vi "参数设置页.vi"() -> ()   [LabVIEW 2016, in "斯坦道CODcr.lvlib"]
uses:
  <vilib>/Plasmionique/MB Master/MB_Master/MB_Master.lvclass
  <vilib>/ptbypt/NI_PtbyPt.lvlib
panel:
  in  "标样核查自动补测":bool caption="通讯连接"
  in  "跨度核查自动补测":bool caption="通讯连接"
  in  "零点核查自动补测":bool caption="通讯连接"
  in  "标样核查标液偏差":dbl caption="标样核查标液偏差："
  in  "跨度核查标液偏差":dbl caption="跨度核查标液偏差："
  in  "零点核查标液偏差":dbl caption="零点核查标液偏差："
  out "低量程上限":dbl caption="低量程上限："
  in  "简易流程路径":path=path "data/流程.xml"
  out "数据刷新时间":string
  in  "通讯连接":bool
  out "MB table":enum32{"Serial", "TCP"}(tab)
  in  "请选择串口:":refnum<visa-resource-name>
  in  "IP":string="127.0.0.1"
  in  "PORT":string="1001"
  in  "通信方式选择":enum16{"串口", "TCP"}(ring)
  in  "盐度自动补偿：":bool
  out "盐度补偿值":dbl caption="盐度补偿值："
  in  "刷新":bool
  in  "测量模式":T1(ring)
  in  "参数下拉列表":u16(ring)
  in  "量程下拉列表":enum16{"低量程", "高量程"}(ring)
  in  "测试流程路径":path=path "data/流程.xml"
  in  "标样核查量程模式":enum16{"高量程", "低量程", "自动"}(ring) caption="标样核查量程模式："
  in  "加标回收量程模式":enum16{"高量程", "低量程", "自动"}(ring) caption="加标回收量程模式："
  in  "跨度核查量程模式":enum16{"高量程", "低量程", "自动"}(ring) caption="跨度核查量程模式："
  in  "零点核查量程模式":enum16{"高量程", "低量程", "自动"}(ring) caption="零点核查量程模式："
  in  "水样测试量程模式":enum16{"高量程", "低量程", "自动"}(ring) caption="水样测试量程模式："
  out "稀释度":dbl caption="稀释度："
  out "阈值（高->低）":dbl caption="阈值（高->低）："
  out "阈值（低->高）":dbl caption="阈值（低->高）："
  out "量程下限":dbl caption="量程下限："
  out "高量程上限":dbl caption="高量程上限："
  out "检出限":dbl caption="检出限："
  out "曲线截距":dbl caption="曲线截距：" format="%#.6f"
  out "曲线斜率":dbl caption="曲线斜率：" format="%#.6f"
  out "二次多项式系数":dbl caption="二次多项式系数：" format="%#.6f"
  out "消解时长":dbl caption="消解时长："
  out "消解温度":dbl caption="消解温度："
  out "测量精度":u16 caption="测量精度："
  in  "标样核查标液浓度":dbl caption="标样核查标液浓度："
  in  "跨度核查标液浓度":dbl caption="跨度核查标液浓度："
  in  "零点核查标液浓度":dbl caption="零点核查标液浓度："
  in  "跨度值":dbl caption="跨度值："
  # "日质控自动补测设置"
  # "mg/L"
  # "mg/L"
  # "±"
  # "mg/L"
  # "%"
  # "mg/L"
  # "%"
  # "mg/L"
  # "ppt"
  # "mg/L"
  # "mg/L"
  # "mg/L"
  # "mg/L"
  # "mg/L"
  # "min"
  # "℃"
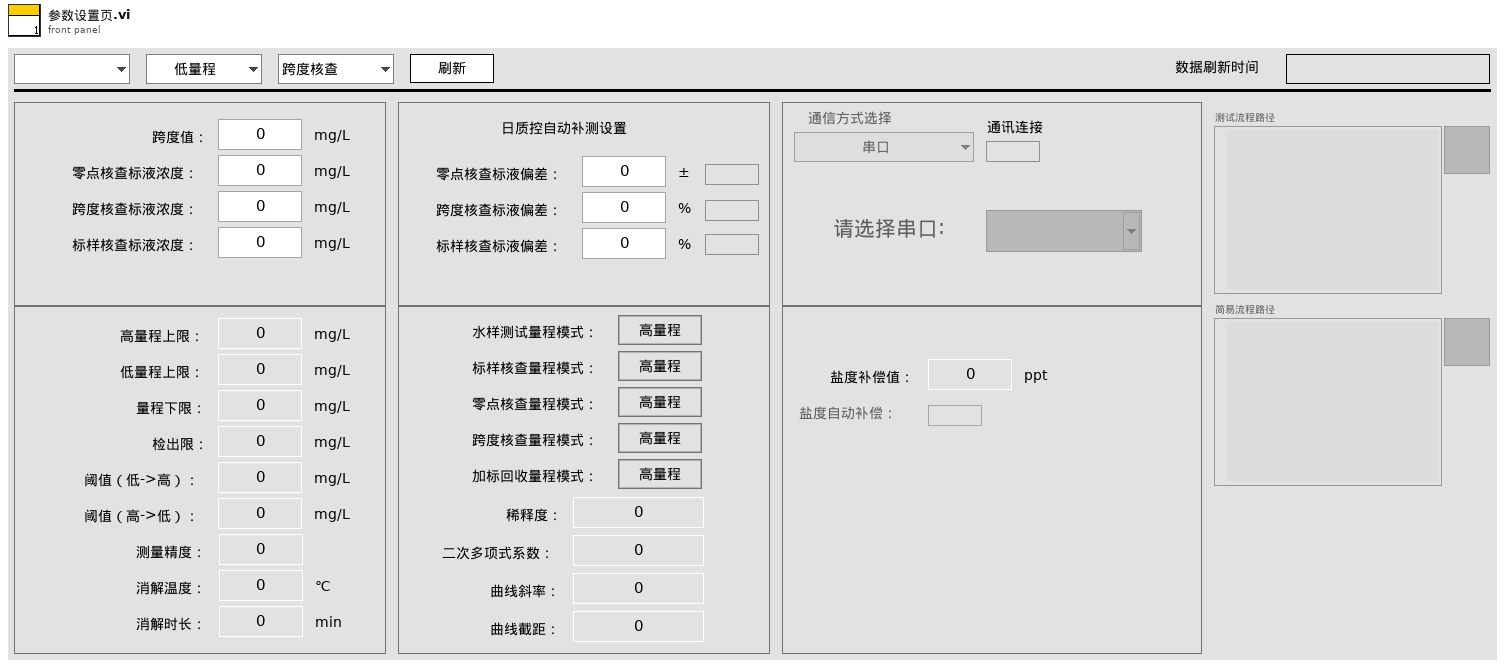
[diagram p1: front panel]
types:
  T1 = enum16{"跨度核查", "水样测量", "零点核查", "标样核查", "加标回收", "快捷测试", "空白校准", "标样校准"}
  T2 = typedef "LVStringsAndValuesArrayTypeDef_U16.ctl" = cluster{"String":string, "Value":u16}[]
  T3 = cluster{"系统时间":timestamp, "工作状态":u16, "测量模式":enum16{"待机", "连续模式", "周期模式", "定点模式", "受控模式", "手动模式"}, "告警代码":u16, "故障代码":u16, "日志代码":u16, "软件版本":u16, "F0":sgl, "F1":sgl, "F2":sgl, "F3":sgl, "T":sgl, "H":sgl, "id":u16, "flowid":u16, "量程":u16, "总磷控温温度1":sgl, "营养盐控温温度2":sgl, "ADC":sgl}
  T4 = enum8{"Enabled", "Disabled", "Disabled and Grayed Out"}
  T5 = cluster{"测量精度":u16, "检出限":dbl, "上限":dbl, "下限":dbl, "阈值（低->高）":dbl, "阈值（高->低）":dbl, "稀释度":dbl}
  T6 = typedef "斯坦道CODcr.lvlib/V3 A版外设参数.ctl" = cluster{"泵类型":u8, "进样速度":u32, "出样速度":u32, "泵阀量":u8, "阀方向":u8, "光谱仪类型":u8, "光谱采样次数":u8, "氙灯次数":u8, "B":u16, "C":u16, "D":u16, "E":u16, "B_COD":u16, "C_COD":u16, "D_COD":u16, "E_COD":u16, "G":u16, "M":u16, "N":u16, "氨氮注射泵控温下限":sgl, "氨氮注射泵控温上限":sgl, "总氮注射泵控温下限":sgl, "总氮注射泵控温上限":sgl, "消解温度下限":sgl, "消解温度上限":sgl, "加热10s限值":sgl, "KP":sgl, "KI":sgl, "KD":sgl, "高温高压阀开阀温度":sgl, "总氮x公式0":u8, "总氮x公式1":sgl, "总氮x公式2":sgl, "总磷浊度稀释系数":sgl, "总磷浊度补偿权重1":sgl, "总磷浊度补偿权重2":sgl, "盐度系数":sgl, "氨氮补偿系数1":sgl, "氨氮补偿系数2":sgl}
  T7 = cluster{"水样测试量程模式":enum16{"高量程", "低量程", "自动"}, "零点核查量程模式":enum16{"高量程", "低量程", "自动"}, "跨度核查量程模式":enum16{"高量程", "低量程", "自动"}, "加标回收量程模式":enum16{"高量程", "低量程", "自动"}, "标样核查量程模式":enum16{"高量程", "低量程", "自动"}}
  T8 = cluster{"总磷跨度值":dbl, "总磷零点标准液浓度":dbl, "总磷跨度标准液浓度":dbl, "总磷标准液标准浓度":dbl, "总氮跨度值":dbl, "总氮零点标准液浓度":dbl, "总氮跨度标准液浓度":dbl, "总氮标准液标准浓度":dbl, "COD跨度值":dbl, "COD零点标准液浓度":dbl, "COD跨度标准液浓度":dbl, "COD标准液标准浓度":dbl, "氨氮跨度值":dbl, "氨氮零点标准液浓度":dbl, "氨氮跨度标准液浓度":dbl, "氨氮标准液标准浓度":dbl, "磷酸盐跨度值":dbl, "磷酸盐零点标准液浓度":dbl, "磷酸盐跨度标准液浓度":dbl, "磷酸盐标准液标准浓度":dbl, "硝氮跨度值":dbl, "硝氮零点标准液浓度":dbl, "硝氮跨度标准液浓度":dbl, "硝氮标准液标准浓度":dbl, "亚硝氮跨度值":dbl, "亚硝氮零点标准液浓度":dbl, "亚硝氮跨度标准液浓度":dbl, "亚硝氮标准液标准浓度":dbl, "硫化物跨度值":dbl, "硫化物零点标准液浓度":dbl, "硫化物跨度标准液浓度":dbl, "硫化物标准液标准浓度":dbl, "硅酸盐跨度值":dbl, "硅酸盐零点标准液浓度":dbl, "硅酸盐跨度标准液浓度":dbl, "硅酸盐标准液标准浓度":dbl, "总磷零点标准液偏差":dbl, "总磷跨度标准液偏差":dbl, "总磷标准液标准偏差":dbl, "总氮零点标准液偏差":dbl, "总氮跨度标准液偏差":dbl, "总氮标准液标准偏差":dbl, "COD零点标准液偏差":dbl, "COD跨度标准液偏差":dbl, "COD标准液标准偏差":dbl, "氨氮零点标准液偏差":dbl, "氨氮跨度标准液偏差":dbl, "氨氮标准液标准偏差":dbl, "磷酸盐零点标准液偏差":dbl, "磷酸盐跨度标准液偏差":dbl, "磷酸盐标准液标准偏差":dbl, "硝氮零点标准液偏差":dbl, "硝氮跨度标准液偏差":dbl, "硝氮标准液标准偏差":dbl, "亚硝氮零点标准液偏差":dbl, "亚硝氮跨度标准液偏差":dbl, "亚硝氮标准液标准偏差":dbl, "硫化物零点标准液偏差":dbl, "硫化物跨度标准液偏差":dbl, "硫化物标准液标准偏差":dbl, "硅酸盐零点标准液偏差":dbl, "硅酸盐跨度标准液偏差":dbl, "硅酸盐标准液标准偏差":dbl, "氟化物跨度值":dbl, "氟化物零点标准液浓度":dbl, "氟化物跨度标准液浓度":dbl, "氟化物标准液标准浓度":dbl, "氟化物零点标准液偏差":dbl, "氟化物跨度标准液偏差":dbl, "氟化物标准液标准偏差":dbl}
  T9 = cluster{"总磷":dbl, "总氮":dbl, "氨氮":dbl, "磷酸盐":dbl, "硝氮":dbl, "亚硝氮":dbl, "硅酸盐":dbl, "硫化物":dbl, "COD":dbl, "氟化物":dbl}
  T10 = cluster{"水样测试量程模式":u16, "零点核查量程模式":u16, "跨度核查量程模式":u16, "加标回收量程模式":u16, "标样核查量程模式":u16}
  T11 = cluster{"水样测试量程模式":enum16{"H", "L", "AUTO"}, "空白核查量程模式":enum16{"H", "L", "AUTO"}, "跨度核查量程模式":enum16{"H", "L", "AUTO"}, "加标回收量程模式":enum16{"H", "L", "AUTO"}, "标样核查量程模式":enum16{"H", "L", "AUTO"}}
  T12 = cluster{"水样测试量程模式":u16, "空白核查量程模式":u16, "跨度核查量程模式":u16, "加标回收量程模式":u16, "标样核查量程模式":u16}
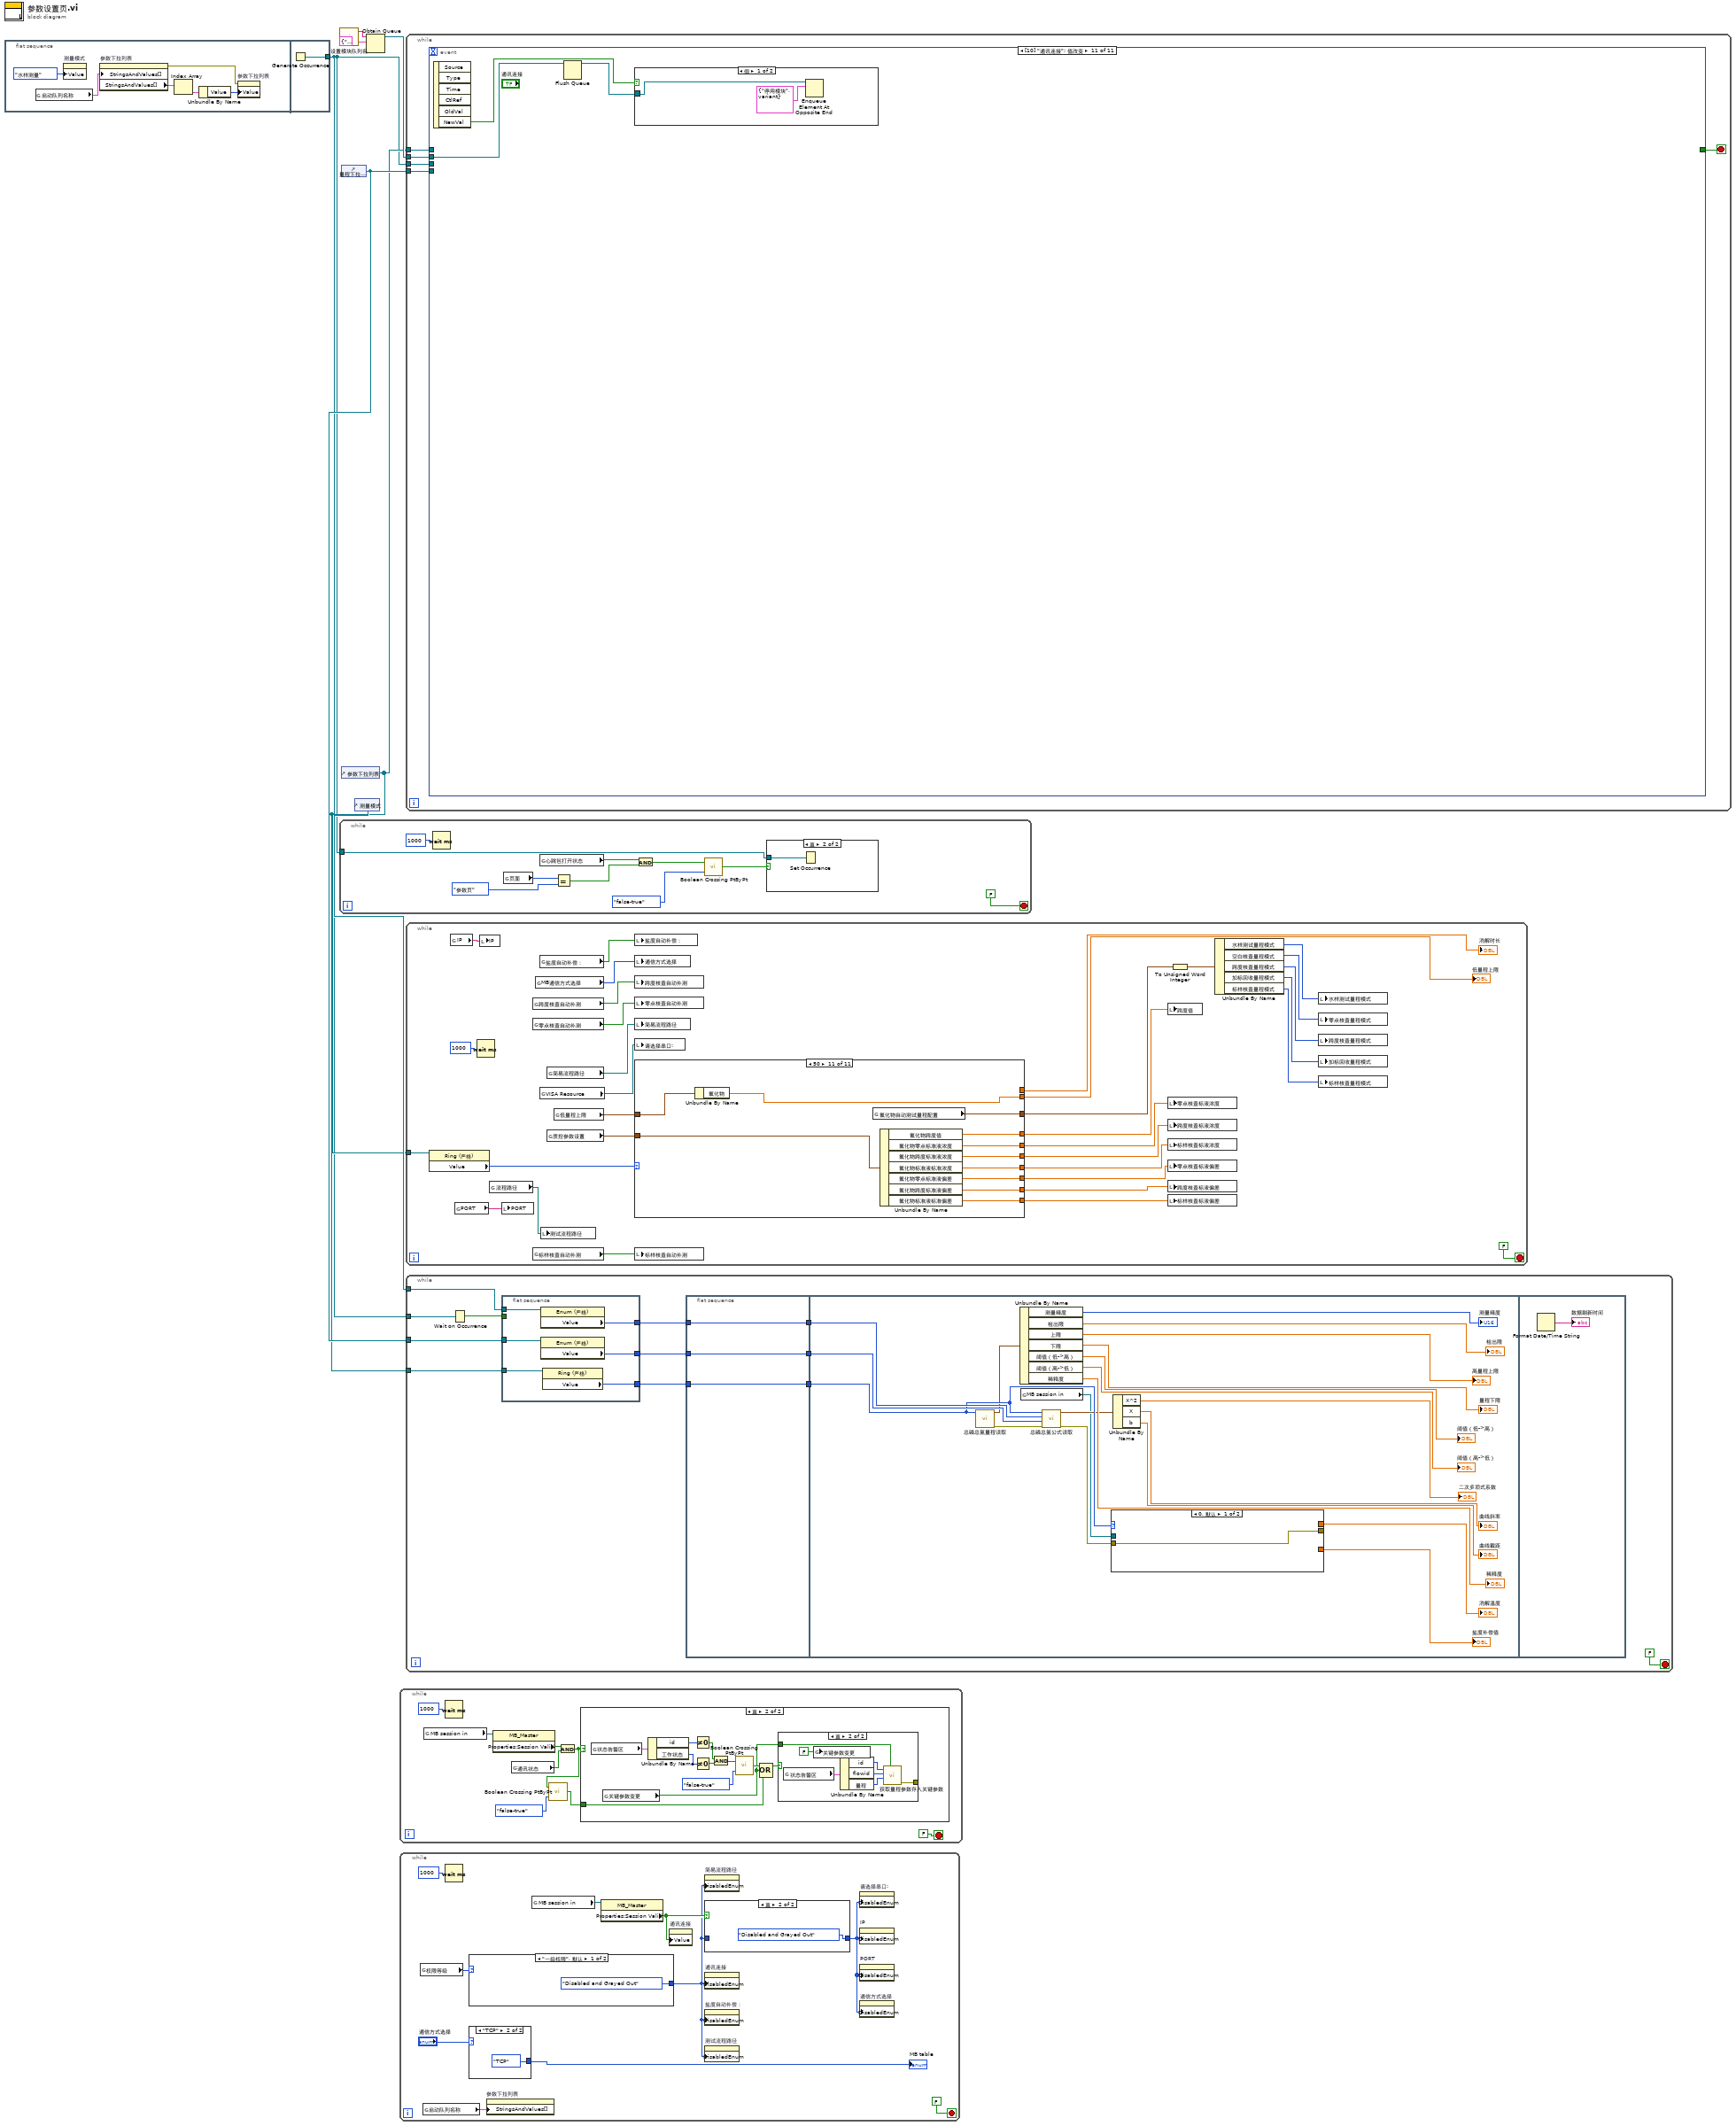
[diagram p0: block diagram]
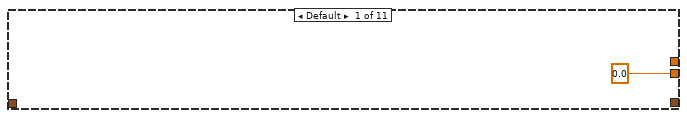
[diagram p5: hidden frame]
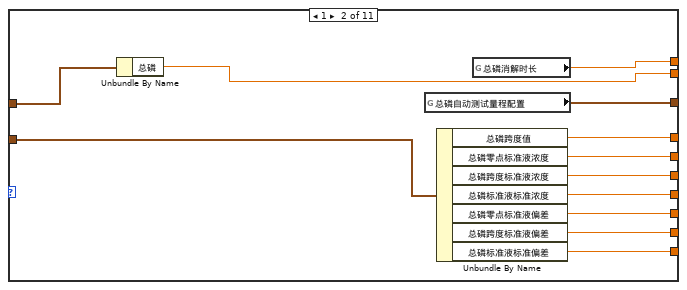
[diagram p6: hidden frame]
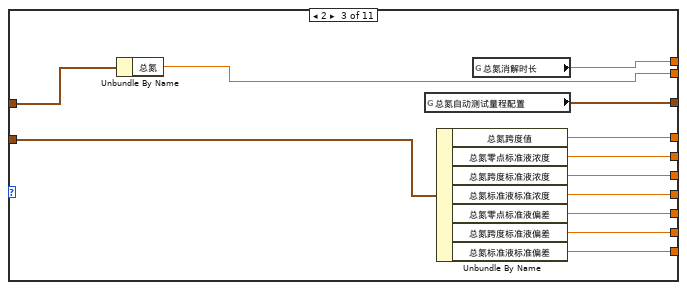
[diagram p7: hidden frame]
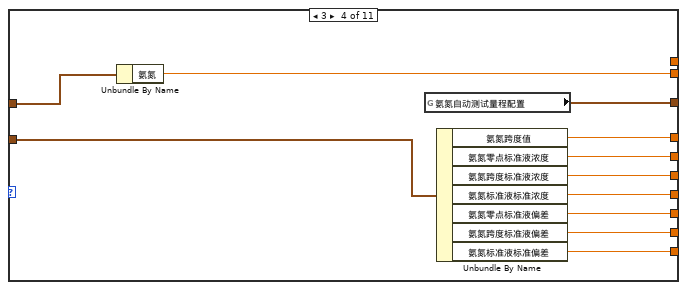
[diagram p8: hidden frame]
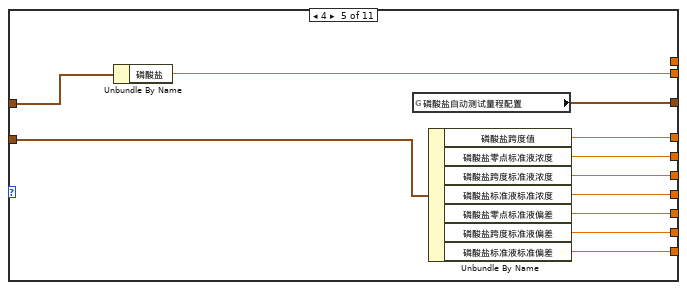
[diagram p9: hidden frame]
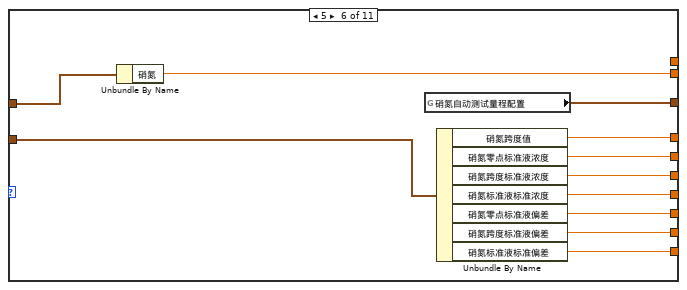
[diagram p10: hidden frame]
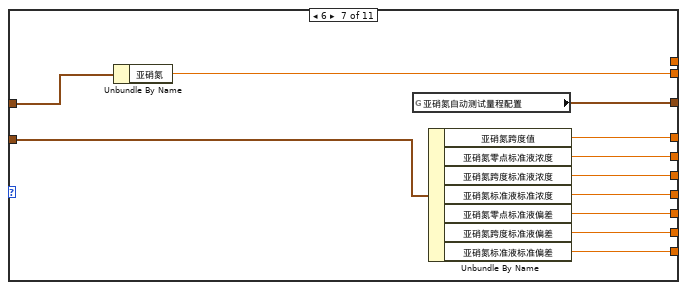
[diagram p11: hidden frame]
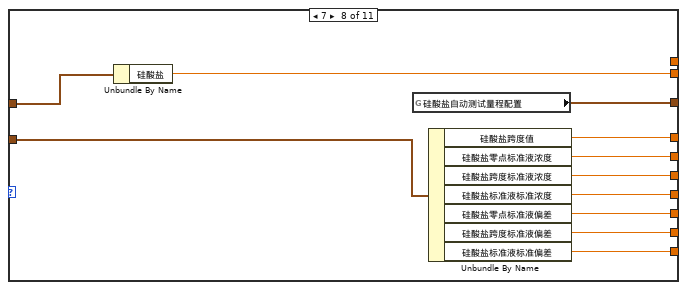
[diagram p12: hidden frame]
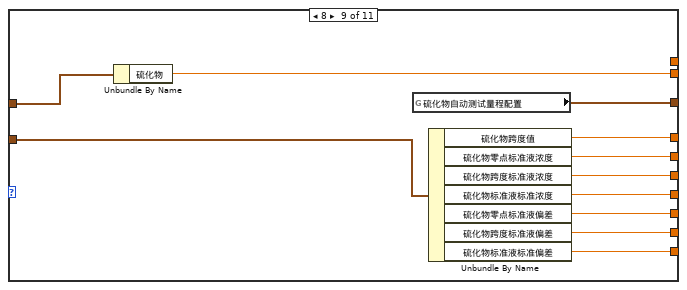
[diagram p13: hidden frame]
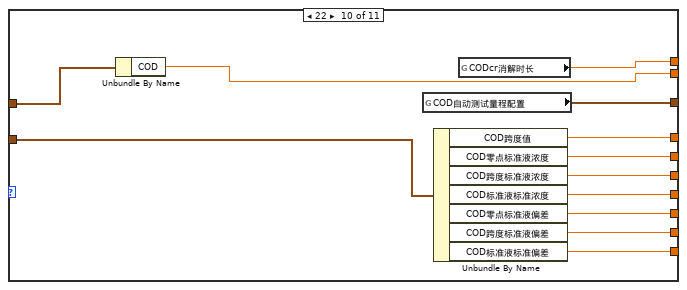
[diagram p14: hidden frame]
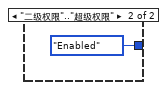
[diagram p15: hidden frame]
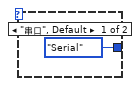
[diagram p16: hidden frame]
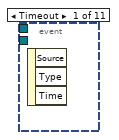
[diagram p18: hidden frame]
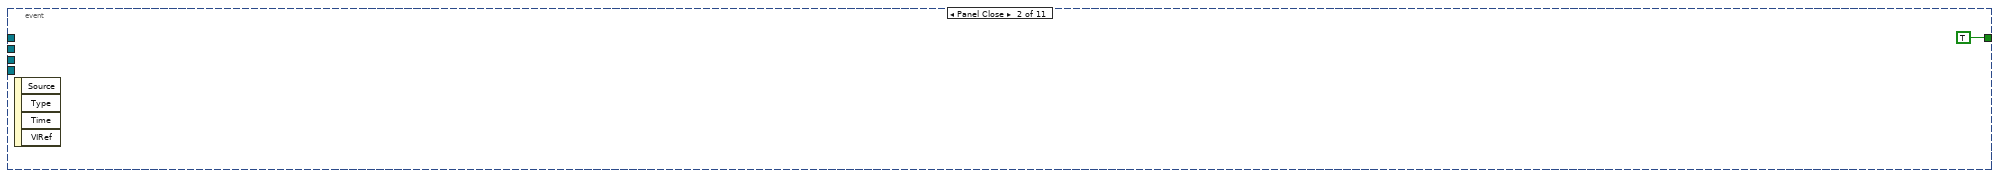
[diagram p19: hidden frame]
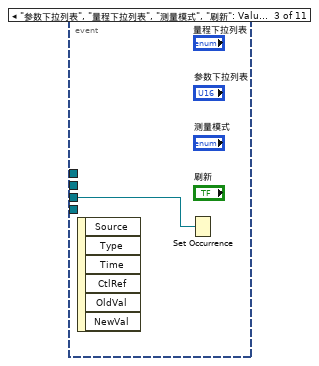
[diagram p20: hidden frame]
diagram:
  n1 = flat-sequence {
    tunnel: [w14] -> w1
    frame #0 {
      n2 = global read "model config var.vi" "启动队列名称"() -> (w9:cluster{"String":string, "Value":u16}[])
      n3 = property on="测量模式" class="Enum (严格)"("Value"=T1."水样测量" ("测量模式")) -> ()  [unwired: 2 in, 2 out]
      n4 = property on="参数下拉列表" class="Ring (严格)"("StringsAndValues[]"=w9) -> (error out=w12:errorcluster, "StringsAndValues[]"=w10:T2)  [unwired: 2 in, 1 out]
      n5 = Index Array(array=w10) -> (element=w11:cluster{"String":string, "Value":u16})  [unwired: 1 in]
      n6 = Unbundle By Name(w11) -> ("Value"=w13:u16)
      n7 = property on="参数下拉列表" class="Ring (严格)"(error in=w12, "Value"=w13) -> ()  [unwired: 1 in, 2 out]
    }
    frame #1 {
      n8 = Generate Occurrence() -> (w14:refnum<k4>)
    }
  }
  n9 = call "设置模块队列名.vi"() -> ("Msg"=w6:string)  [unwired: 5 in]
  n10 = while {
    tunnel: w1 -> [w21]
    stop <- FALSE stop-if-true
    n11 = Wait (ms)(milliseconds to wait=u32 1000 ("等待时间（毫秒）")) -> ()  [unwired: 1 out]
    n12 = global read "VAR总磷总氮全局变量.vi" "页面"() -> (w23:enum16{"主页", "参数页", "校准页"})
    n13 = global read "VAR总磷总氮全局变量.vi" "心跳包打开状态"() -> (w17:bool)
    n14 = Equal?(x=w23, y=enum16{"主页", "参数页", "校准页"}."参数页" ("页面")) -> (x = y?=w22:bool)
    n15 = And(x=w17, y=w22) -> (x .and. y?=w18:bool)
    n16 = call <vilib>:"Boolean Crossing PtByPt.vi"("direction"=enum16{"either", "false-true", "true-false"}."false-true", "input"=w18) -> ("crossing"=w16:bool)  [unwired: 1 in]
    n17 = case shown="真" w16 {
      tunnel: w21 -> [_ w25]
      frame False {
      }
      frame True {
        n18 = Set Occurrence(w25) -> ()
      }
    }
  }
  n19 = control-ref of="量程下拉列表"() -> (w3:refnum<vi>)
  n20 = control-ref of="参数下拉列表"() -> (w2:refnum<vi>)
  n21 = control-ref of="测量模式"() -> (w4:refnum<vi>)
  n22 = Obtain Queue(name (unnamed)=w6, element data type=cluster{"命令":string, "data":variant} {"命令"="", "data"=variant}) -> (queue out=w5:refnum<queue>)  [unwired: 3 in, 2 out]
  n23 = while {
    stop <- FALSE stop-if-true
    n24 = global read "VAR总磷总氮全局变量.vi" "MB session in"() -> (w30:refnum<class "MB_Master.lvclass">)
    n25 = Wait (ms)(milliseconds to wait=u32 1000 ("等待时间（毫秒）")) -> ()  [unwired: 1 out]
    n26 = property class="MB_Master"(reference=w30) -> ("Properties:Session Valid"=w29:bool)  [unwired: 1 in, 2 out]
    n27 = global read "VAR总磷总氮全局变量.vi" "通讯状态"() -> (w32:bool)
    n28 = And(x=w29, y=w32) -> (x .and. y?=w27:bool)
    n29 = call <vilib>:"Boolean Crossing PtByPt.vi"("direction"=enum16{"either", "false-true", "true-false"}."false-true", "input"=w27) -> ("crossing"=w26:bool)  [unwired: 1 in]
    n30 = case shown="真" w27 {
      tunnel: w26 -> [_ w34]
      frame False {
      }
      frame True {
        n31 = global read "VAR总磷总氮全局变量.vi" "状态告警区"() -> (w44:T3)
        n32 = global read "VAR总磷总氮全局变量.vi" "关键参数变更"() -> (w35:bool)
        n33 = Unbundle By Name(w44) -> ("id"=w38:u16, "工作状态"=w43:u16)
        n34 = Not Equal To 0?(x=w38) -> (x != 0?=w39:bool)
        n35 = Not Equal To 0?(x=w43) -> (x != 0?=w40:bool)
        n36 = And(x=w39, y=w40) -> (x .and. y?=w41:bool)
        n37 = call <vilib>:"Boolean Crossing PtByPt.vi"("direction"=enum16{"either", "false-true", "true-false"}."false-true", "input"=w41) -> ("crossing"=w37:bool)  [unwired: 1 in]
        n38 = Compound Arithmetic op=OR ("复合运算")(w37, w35, w34) -> (w36:bool)
        n39 = case shown="真" w36 {
          tunnel: [_ w51] -> _
          tunnel: w35 -> [_ w46]
          frame False {
          }
          frame True {
            n40 = global read "VAR总磷总氮全局变量.vi" "状态告警区"() -> (w50:T3)
            n41 = global write "VAR总磷总氮全局变量.vi" "关键参数变更"(FALSE ("关键参数变更")) -> ()
            n42 = Unbundle By Name(w50) -> ("id"=w49:u16, "flowid"=w48:u16, "量程"=w47:u16)
            n43 = call "获取量程参数存入关键参数.vi"("关键参数变更"=w46, "量程"=w47, "flowid"=w48, "id"=w49) -> ("error out"=w51:errorcluster)  [unwired: 7 in]
          }
        }
      }
    }
  }
  n44 = while {
    stop <- FALSE stop-if-true
    n45 = global read "VAR总磷总氮全局变量.vi" "权限等级"() -> (w54:enum16{"一级权限", "二级权限", "三级权限", "超级权限"})
    n46 = global read "model config var.vi" "启动队列名称"() -> (w52:cluster{"String":string, "Value":u16}[])
    n47 = Wait (ms)(milliseconds to wait=u32 1000 ("等待时间（毫秒）")) -> ()  [unwired: 1 out]
    n48 = case shown="\"一级权限\", 默认" w54 {
      tunnel: [T4."Disabled and Grayed Out" ("禁用") T4."Enabled" ("禁用")] -> w53
      frame "一级权限", Default {
      }
      frame "二级权限".."超级权限" {
      }
    }
    n49 = case shown="\"TCP\"" "通信方式选择" {
      tunnel: [enum32{"Serial", "TCP"}."Serial" ("MB table") enum32{"Serial", "TCP"}."TCP" ("MB table")] -> w56
      frame "串口", Default {
      }
      frame "TCP" {
      }
    }
    "MB table" <- w56
    n50 = property on="参数下拉列表" class="Ring (严格)"("StringsAndValues[]"=w52) -> ()  [unwired: 2 in, 2 out]
    n51 = global read "VAR总磷总氮全局变量.vi" "MB session in"() -> (w60:refnum<class "MB_Master.lvclass">)
    n52 = property class="MB_Master"(reference=w60) -> ("Properties:Session Valid"=w58:bool)  [unwired: 1 in, 2 out]
    n53 = property on="通讯连接" class="Bool (严格)"("Value"=w58) -> ()  [unwired: 2 in, 2 out]
    n54 = property on="简易流程路径" class="Path"("DisabledEnum"=w53) -> ()  [unwired: 2 in, 2 out]
    n55 = case shown="真" w58 {
      tunnel: [w66 T4."Disabled and Grayed Out" ("禁用")] -> w57
      tunnel: w53 -> [w66 _]
      frame False {
      }
      frame True {
      }
    }
    n56 = property on="通讯连接" class="Bool (严格)"("DisabledEnum"=w53) -> ()  [unwired: 2 in, 2 out]
    n57 = property on="盐度自动补偿：" class="Bool (严格)"("DisabledEnum"=w53) -> ()  [unwired: 2 in, 2 out]
    n58 = property on="测试流程路径" class="Path"("DisabledEnum"=w53) -> ()  [unwired: 2 in, 2 out]
    n59 = property on="请选择串口:" class="VISAName"("DisabledEnum"=w57) -> ()  [unwired: 2 in, 2 out]
    n60 = property on="IP" class="Str"("DisabledEnum"=w57) -> ()  [unwired: 2 in, 2 out]
    n61 = property on="PORT" class="Str"("DisabledEnum"=w57) -> ()  [unwired: 2 in, 2 out]
    n62 = property on="通信方式选择" class="Enum (严格)"("DisabledEnum"=w57) -> ()  [unwired: 2 in, 2 out]
  }
  n63 = while {
    tunnel: w1 -> [w71]
    tunnel: w2 -> [w70]
    tunnel: w5 -> [w69]
    tunnel: w3 -> [w68]
    stop <- w72 stop-if-true
    n64 = event shown="[10] \"通讯连接\": 值改变" {
      selector: _ -> [_ _ _ _ _ _ _ _ _ _ _]
      dyn-events: _ -> [_ _ _ _ _ _ _ _ _ _ _]
      timeout: _ -> [_ _ _ _ _ _ _ _ _ _ _]
      tunnel: [_ TRUE _ _ _ _ _ _ _ _ _] -> w72
      tunnel: w71 -> [_ _ w74 _ _ _ _ _ _ w122 _]
      tunnel: w70 -> [_ _ _ _ w93 _ _ _ _ w124 _]
      tunnel: w69 -> [_ _ _ _ _ _ _ _ _ _ w293]
      tunnel: w68 -> [_ _ _ _ _ _ _ _ _ _ _]
      event Timeout {
        n65 = event-data() -> ()  [unwired: 1 in, 3 out]
      }
      event Panel Close {
        n66 = event-data() -> ()  [unwired: 1 in, 4 out]
      }
      event "参数下拉列表", "量程下拉列表", "测量模式", "刷新": Value Change {
        n67 = event-data() -> ()  [unwired: 1 in, 6 out]
        n68 = Set Occurrence(w74) -> ()
      }
      event "跨度值", "零点核查标液浓度", "跨度核查标液浓度", "标样核查标液浓度", "消解温度", "消解时长", "检出限", "高量程上限", "量程下限", "阈值（低->高）", "阈值（高->低）", "稀释度", "低量程上限", "零点核查标液偏差", "跨度核查标液偏差", "标样核查标液偏差": Mouse Down {
        n69 = event-data() -> ("CtlRef"=w76:refnum<vi>)  [unwired: 1 in, 5 out]
        n70 = global read "VAR总磷总氮全局变量.vi" "权限等级"() -> (w75:enum16{"一级权限", "二级权限", "三级权限", "超级权限"})
        n71 = case shown="\"二级权限\"..\"超级权限\"" w75 {
          tunnel: w76 -> [_ w80]
          frame "一级权限", Default {
          }
          frame "二级权限".."超级权限" {
            n72 = property class="DigNum (严格)"(reference=w80) -> (reference out=w78:refnum<vi>, "Value"=w79:dbl)  [unwired: 1 in, 1 out]
            n73 = call "数字键盘.vi"("OldNumber"=w79) -> ("NewNumber"=w77:dbl)
            n74 = property class="DigNum (严格)"(reference=w78, "Val(Sgnl)"=w77) -> ()  [unwired: 1 in, 2 out]
          }
        }
      }
      event "测量精度", "检出限", "高量程上限", "量程下限", "阈值（低->高）", "阈值（高->低）", "稀释度": Value Change {
        n75 = event-data() -> ()  [unwired: 1 in, 6 out]
        n76 = property class="Ring (严格)"(reference=w93) -> ("Value"=w92:u16)  [unwired: 1 in, 2 out]
        n77 = local read "阈值（低->高）"() -> (w86:dbl)
        n78 = local read "阈值（高->低）"() -> (w85:dbl)
        n79 = local read "高量程上限"() -> (w89:dbl)
        n80 = local read "测量精度"() -> (w83:u16)
        n81 = local read "量程下限"() -> (w88:dbl)
        n82 = local read "检出限"() -> (w87:dbl)
        n83 = local read "稀释度"() -> (w84:dbl)
        n84 = Bundle By Name(cluster=T5 {"测量精度"=0, "检出限"=0.0, "上限"=0.0, "下限"=0.0, "阈值（低->高）"=0.0, "阈值（高->低）"=0.0, "稀释度"=0.0} ("量程参数写入"), "测量精度"=w83, "检出限"=w87, "上限"=w89, "下限"=w88, "阈值（低->高）"=w86, "阈值（高->低）"=w85, "稀释度"=w84) -> (w90:T5)
        n85 = call "总磷总氮量程写入.vi"("量程参数写入"=w90, "测量参数"=w92) -> ("error out"=w81:errorcluster)  [unwired: 8 in]
        n86 = case shown="无错误" w81 {
          tunnel: ["写入成功" "写入失败"] -> w82
          frame No Error {
            n87 = global write "VAR总磷总氮全局变量.vi" "关键参数变更"(TRUE ("关键参数变更")) -> ()
          }
          frame Error {
          }
        }
        n88 = One Button Dialog(message=w82) -> ()  [unwired: 1 in, 1 out]
      }
      event "消解温度": Value Change {
        n89 = event-data() -> ("NewVal"=w99:dbl)  [unwired: 1 in, 5 out]
        n90 = global read "VAR总磷总氮全局变量.vi" "MB session in"() -> (w100:refnum<class "MB_Master.lvclass">)
        n91 = call "读取外设配置.vi"("MB session in"=w100) -> ("error out"=w103:errorcluster, "外设配置"=w102:T6)  [unwired: 8 in, 1 out]
        n92 = Bundle By Name(cluster=w102, "消解温度下限"=w99) -> (w101:T6)
        n93 = call "写入外设配置.vi"("error in (no error)"=w103, "外设配置"=w101, "MB session in"=w100) -> ("error out"=w98:errorcluster)  [unwired: 7 in, 1 out]
        n94 = case shown="错误" w98 {
          tunnel: ["写入成功" "写入失败"] -> w97
          frame No Error {
          }
          frame Error {
          }
        }
        n95 = One Button Dialog(message=w97) -> ()  [unwired: 1 in, 1 out]
      }
      event "测量精度": Mouse Down {
        n96 = event-data() -> ("CtlRef"=w107:refnum<vi>)  [unwired: 1 in, 7 out]
        n97 = global read "VAR总磷总氮全局变量.vi" "权限等级"() -> (w106:enum16{"一级权限", "二级权限", "三级权限", "超级权限"})
        n98 = case shown="\"二级权限\"..\"超级权限\"" w106 {
          tunnel: w107 -> [_ w111]
          frame "一级权限", Default {
          }
          frame "二级权限".."超级权限" {
            n99 = property class="DigNum (严格)"(reference=w111) -> (reference out=w109:refnum<vi>, "Value"=w110:u16)  [unwired: 1 in, 1 out]
            n100 = call "数字键盘.vi"("OldNumber"=w110) -> ("NewNumber"=w108:dbl)
            n101 = property class="DigNum (严格)"(reference=w109, "Val(Sgnl)"=w108) -> ()  [unwired: 1 in, 2 out]
          }
        }
      }
      event "盐度补偿值": Mouse Down {
        n102 = event-data() -> ("CtlRef"=w113:refnum<vi>)  [unwired: 1 in, 3 out]
        n103 = global read "VAR总磷总氮全局变量.vi" "权限等级"() -> (w112:enum16{"一级权限", "二级权限", "三级权限", "超级权限"})
        n104 = case shown="\"二级权限\"..\"超级权限\"" w112 {
          tunnel: w113 -> [_ w115]
          frame "一级权限", Default {
          }
          frame "二级权限".."超级权限" {
            n105 = case shown="假" "盐度自动补偿：" {
              tunnel: w115 -> [w119 _]
              frame False {
                n106 = property class="DigNum (严格)"(reference=w119) -> (reference out=w117:refnum<vi>, "Value"=w118:dbl)  [unwired: 1 in, 1 out]
                n107 = call "数字键盘.vi"("OldNumber"=w118) -> ("NewNumber"=w116:dbl)
                n108 = property class="DigNum (严格)"(reference=w117, "Val(Sgnl)"=w116) -> ()  [unwired: 1 in, 2 out]
              }
              frame True {
              }
            }
          }
        }
      }
      event "盐度补偿值": Value Change {
        n109 = event-data() -> ("NewVal"=w120:dbl)  [unwired: 1 in, 5 out]
        n110 = global read "VAR总磷总氮全局变量.vi" "MB session in"() -> (w121:refnum<class "MB_Master.lvclass">)
        n111 = call "盐度补偿值写入.vi"("盐度补偿值"=w120, "MB session in"=w121) -> ()  [unwired: 8 in, 2 out]
      }
      event "跨度值", "零点核查标液浓度", "跨度核查标液浓度", "标样核查标液浓度", "消解时长", "水样测试量程模式", "零点核查量程模式", "跨度核查量程模式", "加标回收量程模式", "标样核查量程模式", "测试流程路径", "盐度自动补偿：", "IP", "PORT", "请选择串口:", "通信方式选择", "简易流程路径", "低量程上限", "零点核查标液偏差", "跨度核查标液偏差", "标样核查标液偏差", "零点核查自动补测", "跨度核查自动补测", "标样核查自动补测": Value Change {
        n112 = event-data() -> ()  [unwired: 1 in, 6 out]
        n113 = global read "VAR总磷总氮全局变量.vi" "权限等级"() -> (w123:enum16{"一级权限", "二级权限", "三级权限", "超级权限"})
        n114 = case shown="\"二级权限\"..\"超级权限\"" w123 {
          tunnel: w124 -> [_ w126]
          tunnel: w122 -> [w125 _]
          frame "一级权限", Default {
            n115 = Set Occurrence(w125) -> ()
          }
          frame "二级权限".."超级权限" {
            n116 = flat-sequence {
              tunnel: w126 -> [w156]
              frame #0 {
                n117 = property class="Ring (严格)"(reference=w156) -> ("Value"=w155:u16)  [unwired: 1 in, 2 out]
                n118 = global write "总磷总氮断电保存全局变量.vi" "IP"("IP") -> ()
                n119 = global write "总磷总氮断电保存全局变量.vi" "PORT"("PORT") -> ()
                n120 = local read "盐度自动补偿："() -> (w142:bool)
                n121 = local read "通信方式选择"() -> (w138:enum16{"串口", "TCP"})
                n122 = global write "总磷总氮断电保存全局变量.vi" "流程路径"("测试流程路径") -> ()
                n123 = global write "总磷总氮断电保存全局变量.vi" "简易流程路径"("简易流程路径") -> ()
                n124 = global write "总磷总氮断电保存全局变量.vi" "VISA Resource"("请选择串口:") -> ()
                n125 = global write "总磷总氮断电保存全局变量.vi" "MB通信方式选择"(w138) -> ()
                n126 = global write "总磷总氮断电保存全局变量.vi" "盐度自动补偿："(w142) -> ()
                n127 = global write "总磷总氮断电保存全局变量.vi" "标样核查自动补测"("标样核查自动补测") -> ()
                n128 = global write "总磷总氮断电保存全局变量.vi" "跨度核查自动补测"("跨度核查自动补测") -> ()
                n129 = global write "总磷总氮断电保存全局变量.vi" "零点核查自动补测"("零点核查自动补测") -> ()
                n130 = Bundle("水样测试量程模式"="水样测试量程模式", "零点核查量程模式"="零点核查量程模式", "跨度核查量程模式"="跨度核查量程模式", "加标回收量程模式"="加标回收量程模式", "标样核查量程模式"="标样核查量程模式") -> (w144:T7)  [unwired: 1 in]
                n131 = global read "总磷总氮断电保存全局变量.vi" "质控参数设置"() -> (w150:T8)
                n132 = global read "总磷总氮断电保存全局变量.vi" "低量程上限"() -> (w135:T9)
                n133 = local read "消解时长"() -> (w137:dbl)
                n134 = property on="低量程上限" class="DigNum (严格)"() -> ("Value"=w133:dbl)  [unwired: 2 in, 2 out]
                n135 = To Unsigned Word Integer(number=w144) -> (unsigned 16bit integer=w143:T10)
                n136 = case shown="50" w155 {
                  tunnel: "跨度值" -> [_ w170 w184 w197 w210 w223 w236 w249 w262 w276 w289]
                  tunnel: "标样核查标液浓度" -> [_ w167 w181 w194 w207 w220 w233 w246 w259 w273 w286]
                  tunnel: "跨度核查标液浓度" -> [_ w168 w182 w195 w208 w221 w234 w247 w260 w274 w287]
                  tunnel: "零点核查标液浓度" -> [_ w169 w183 w196 w209 w222 w235 w248 w261 w275 w288]
                  tunnel: w150 -> [_ w172 w186 w199 w212 w225 w238 w251 w264 w278 w291]
                  tunnel: w143 -> [_ w166 w180 w193 w206 w219 w232 w245 w258 w271 w285]
                  tunnel: w137 -> [_ w165 w179 _ _ _ _ _ _ w272 _]
                  tunnel: w135 -> [w158 w163 w178 w192 w205 w218 w231 w244 w257 w270 w284]
                  tunnel: [w158 w162 w176 w191 w204 w217 w230 w243 w256 w269 w283] -> w134
                  tunnel: w133 -> [_ w164 w177 w190 w203 w216 w229 w242 w255 w268 w282]
                  tunnel: "标样核查标液偏差" -> [_ w161 w173 w187 w200 w215 w226 w239 w252 w265 w279]
                  tunnel: "跨度核查标液偏差" -> [_ w160 w174 w188 w201 w214 w227 w240 w253 w266 w280]
                  tunnel: "零点核查标液偏差" -> [_ w159 w175 w189 w202 w213 w228 w241 w254 w267 w281]
                  frame 0, Default {
                  }
                  frame 1 {
                    n137 = global write "总磷总氮断电保存全局变量.vi" "总磷消解时长"(w165) -> ()
                    n138 = global write "总磷总氮断电保存全局变量.vi" "总磷自动测试量程配置"(w166) -> ()
                    n139 = Bundle By Name(cluster=w172, "总磷跨度值"=w170, "总磷零点标准液浓度"=w169, "总磷跨度标准液浓度"=w168, "总磷标准液标准浓度"=w167, "总磷零点标准液偏差"=w159, "总磷跨度标准液偏差"=w160, "总磷标准液标准偏差"=w161) -> (w171:T8)
                    n140 = Bundle By Name(cluster=w163, "总磷"=w164) -> (w162:T9)
                    n141 = global write "总磷总氮断电保存全局变量.vi" "质控参数设置"(w171) -> ()
                  }
                  frame 2 {
                    n142 = global write "总磷总氮断电保存全局变量.vi" "总氮消解时长"(w179) -> ()
                    n143 = global write "总磷总氮断电保存全局变量.vi" "总氮自动测试量程配置"(w180) -> ()
                    n144 = Bundle By Name(cluster=w186, "总氮跨度值"=w184, "总氮零点标准液浓度"=w183, "总氮跨度标准液浓度"=w182, "总氮标准液标准浓度"=w181, "总氮零点标准液偏差"=w175, "总氮跨度标准液偏差"=w174, "总氮标准液标准偏差"=w173) -> (w185:T8)
                    n145 = Bundle By Name(cluster=w178, "总氮"=w177) -> (w176:T9)
                    n146 = global write "总磷总氮断电保存全局变量.vi" "质控参数设置"(w185) -> ()
                  }
                  frame 3 {
                    n147 = global write "总磷总氮断电保存全局变量.vi" "氨氮自动测试量程配置"(w193) -> ()
                    n148 = Bundle By Name(cluster=w199, "氨氮跨度值"=w197, "氨氮零点标准液浓度"=w196, "氨氮跨度标准液浓度"=w195, "氨氮标准液标准浓度"=w194, "氨氮零点标准液偏差"=w189, "氨氮跨度标准液偏差"=w188, "氨氮标准液标准偏差"=w187) -> (w198:T8)
                    n149 = Bundle By Name(cluster=w192, "氨氮"=w190) -> (w191:T9)
                    n150 = global write "总磷总氮断电保存全局变量.vi" "质控参数设置"(w198) -> ()
                  }
                  frame 4 {
                    n151 = Bundle By Name(cluster=w212, "磷酸盐跨度值"=w210, "磷酸盐零点标准液浓度"=w209, "磷酸盐跨度标准液浓度"=w208, "磷酸盐标准液标准浓度"=w207, "磷酸盐零点标准液偏差"=w202, "磷酸盐跨度标准液偏差"=w201, "磷酸盐标准液标准偏差"=w200) -> (w211:T8)
                    n152 = global write "总磷总氮断电保存全局变量.vi" "磷酸盐自动测试量程配置"(w206) -> ()
                    n153 = Bundle By Name(cluster=w205, "磷酸盐"=w203) -> (w204:T9)
                    n154 = global write "总磷总氮断电保存全局变量.vi" "质控参数设置"(w211) -> ()
                  }
                  frame 5 {
                    n155 = global write "总磷总氮断电保存全局变量.vi" "硝氮自动测试量程配置"(w219) -> ()
                    n156 = Bundle By Name(cluster=w225, "硝氮跨度值"=w223, "硝氮零点标准液浓度"=w222, "硝氮跨度标准液浓度"=w221, "硝氮标准液标准浓度"=w220, "硝氮零点标准液偏差"=w213, "硝氮跨度标准液偏差"=w214, "硝氮标准液标准偏差"=w215) -> (w224:T8)
                    n157 = Bundle By Name(cluster=w218, "硝氮"=w216) -> (w217:T9)
                    n158 = global write "总磷总氮断电保存全局变量.vi" "质控参数设置"(w224) -> ()
                  }
                  frame 6 {
                    n159 = Bundle By Name(cluster=w238, "亚硝氮跨度值"=w236, "亚硝氮零点标准液浓度"=w235, "亚硝氮跨度标准液浓度"=w234, "亚硝氮标准液标准浓度"=w233, "亚硝氮零点标准液偏差"=w228, "亚硝氮跨度标准液偏差"=w227, "亚硝氮标准液标准偏差"=w226) -> (w237:T8)
                    n160 = global write "总磷总氮断电保存全局变量.vi" "亚硝氮自动测试量程配置"(w232) -> ()
                    n161 = Bundle By Name(cluster=w231, "亚硝氮"=w229) -> (w230:T9)
                    n162 = global write "总磷总氮断电保存全局变量.vi" "质控参数设置"(w237) -> ()
                  }
                  frame 7 {
                    n163 = Bundle By Name(cluster=w251, "硅酸盐跨度值"=w249, "硅酸盐零点标准液浓度"=w248, "硅酸盐跨度标准液浓度"=w247, "硅酸盐标准液标准浓度"=w246, "硅酸盐零点标准液偏差"=w241, "硅酸盐跨度标准液偏差"=w240, "硅酸盐标准液标准偏差"=w239) -> (w250:T8)
                    n164 = global write "总磷总氮断电保存全局变量.vi" "硅酸盐自动测试量程配置"(w245) -> ()
                    n165 = Bundle By Name(cluster=w244, "硅酸盐"=w242) -> (w243:T9)
                    n166 = global write "总磷总氮断电保存全局变量.vi" "质控参数设置"(w250) -> ()
                  }
                  frame 8 {
                    n167 = Bundle By Name(cluster=w264, "硫化物跨度值"=w262, "硫化物零点标准液浓度"=w261, "硫化物跨度标准液浓度"=w260, "硫化物标准液标准浓度"=w259, "硫化物零点标准液偏差"=w254, "硫化物跨度标准液偏差"=w253, "硫化物标准液标准偏差"=w252) -> (w263:T8)
                    n168 = global write "总磷总氮断电保存全局变量.vi" "硫化物自动测试量程配置"(w258) -> ()
                    n169 = Bundle By Name(cluster=w257, "硫化物"=w255) -> (w256:T9)
                    n170 = global write "总磷总氮断电保存全局变量.vi" "质控参数设置"(w263) -> ()
                  }
                  frame 22 {
                    n171 = global write "总磷总氮断电保存全局变量.vi" "CODcr消解时长"(w272) -> ()
                    n172 = global write "总磷总氮断电保存全局变量.vi" "COD自动测试量程配置"(w271) -> ()
                    n173 = Bundle By Name(cluster=w278, "COD跨度值"=w276, "COD零点标准液浓度"=w275, "COD跨度标准液浓度"=w274, "COD标准液标准浓度"=w273, "COD零点标准液偏差"=w267, "COD跨度标准液偏差"=w266, "COD标准液标准偏差"=w265) -> (w277:T8)
                    n174 = Bundle By Name(cluster=w270, "COD"=w268) -> (w269:T9)
                    n175 = global write "总磷总氮断电保存全局变量.vi" "质控参数设置"(w277) -> ()
                  }
                  frame 50 {
                    n176 = global write "总磷总氮断电保存全局变量.vi" "氟化物自动测试量程配置"(w285) -> ()
                    n177 = Bundle By Name(cluster=w291, "氟化物跨度值"=w289, "氟化物零点标准液浓度"=w288, "氟化物跨度标准液浓度"=w287, "氟化物标准液标准浓度"=w286, "氟化物零点标准液偏差"=w281, "氟化物跨度标准液偏差"=w280, "氟化物标准液标准偏差"=w279) -> (w290:T8)
                    n178 = Bundle By Name(cluster=w284, "氟化物"=w282) -> (w283:T9)
                    n179 = global write "总磷总氮断电保存全局变量.vi" "质控参数设置"(w290) -> ()
                  }
                }
                n180 = global write "总磷总氮断电保存全局变量.vi" "低量程上限"(w134) -> ()
              }
              frame #1 {
                n181 = call "仪器配置写入.vi"() -> ()  [unwired: 11 in, 1 out]
              }
            }
          }
        }
      }
      event "通讯连接": Value Change {
        n182 = event-data() -> ("NewVal"=w292:bool)  [unwired: 1 in, 5 out]
        n183 = Flush Queue(queue=w293) -> (queue out=w294:refnum<queue>)  [unwired: 1 in, 2 out]
        n184 = case shown="假" w292 {
          tunnel: w294 -> [w295 w297]
          frame False {
            n185 = Enqueue Element At Opposite End(queue=w295, element=cluster{"命令":string, "data":variant} {"命令"="停用模块", "data"=variant} ("元素")) -> ()  [unwired: 2 in, 3 out]
          }
          frame True {
            n186 = Enqueue Element At Opposite End(queue=w297, element=cluster{"命令":string, "data":variant} {"命令"="启用模块", "data"=variant} ("元素")) -> ()  [unwired: 2 in, 3 out]
          }
        }
      }
    }
  }
  n187 = while {
    tunnel: w2 -> [w309]
    stop <- FALSE stop-if-true
    n188 = property class="Ring (严格)"(reference=w309) -> ("Value"=w308:u16)  [unwired: 1 in, 2 out]
    n189 = global read "总磷总氮断电保存全局变量.vi" "IP"() -> (w326:string)
    n190 = global read "总磷总氮断电保存全局变量.vi" "PORT"() -> (w327:string)
    n191 = Wait (ms)(milliseconds to wait=u32 1000 ("等待时间（毫秒）")) -> ()  [unwired: 1 out]
    n192 = local write "IP"(w326) -> ()
    n193 = global read "总磷总氮断电保存全局变量.vi" "流程路径"() -> (w325:path)
    n194 = local write "PORT"(w327) -> ()
    n195 = global read "总磷总氮断电保存全局变量.vi" "跨度核查自动补测"() -> (w299:bool)
    n196 = global read "总磷总氮断电保存全局变量.vi" "零点核查自动补测"() -> (w301:bool)
    n197 = global read "总磷总氮断电保存全局变量.vi" "标样核查自动补测"() -> (w300:bool)
    n198 = global read "总磷总氮断电保存全局变量.vi" "MB通信方式选择"() -> (w323:enum16{"串口", "TCP"})
    n199 = global read "总磷总氮断电保存全局变量.vi" "盐度自动补偿："() -> (w324:bool)
    n200 = global read "总磷总氮断电保存全局变量.vi" "VISA Resource"() -> (w328:refnum<visa-resource-name>)
    n201 = local write "测试流程路径"(w325) -> ()
    n202 = global read "总磷总氮断电保存全局变量.vi" "简易流程路径"() -> (w307:path)
    n203 = global read "总磷总氮断电保存全局变量.vi" "质控参数设置"() -> (w318:T8)
    n204 = global read "总磷总氮断电保存全局变量.vi" "低量程上限"() -> (w306:T9)
    n205 = local write "盐度自动补偿："(w324) -> ()
    n206 = local write "通信方式选择"(w323) -> ()
    n207 = local write "跨度核查自动补测"(w299) -> ()
    n208 = local write "零点核查自动补测"(w301) -> ()
    n209 = local write "简易流程路径"(w307) -> ()
    n210 = local write "请选择串口:"(w328) -> ()
    n211 = case shown="50" w308 {
      tunnel: [_ w343 w355 w366 w377 w388 w399 w410 w421 w433 w444] -> w316
      tunnel: [_ w342 w354 _ _ _ _ _ _ w432 _] -> w317
      tunnel: w318 -> [_ w341 w353 w365 w376 w387 w398 w409 w420 w431 w443]
      tunnel: [_ w340 w352 w364 w375 w386 w397 w408 w419 w430 w442] -> w319
      tunnel: [_ w339 w351 w363 w374 w385 w396 w407 w418 w429 w441] -> w320
      tunnel: [_ w338 w350 w362 w373 w384 w395 w406 w417 w428 w440] -> w321
      tunnel: [_ w337 w349 w361 w372 w383 w394 w405 w416 w427 w439] -> w322
      tunnel: w306 -> [_ w336 w348 w360 w371 w382 w393 w404 w415 w426 w438]
      tunnel: [0.0 ("COD") w335 w347 w359 w370 w381 w392 w403 w414 w425 w437] -> w305
      tunnel: [_ w334 w346 w358 w369 w380 w391 w402 w413 w424 w436] -> w304
      tunnel: [_ w333 w345 w357 w368 w379 w390 w401 w412 w423 w435] -> w303
      tunnel: [_ w332 w344 w356 w367 w378 w389 w400 w411 w422 w434] -> w302
      frame Default {
      }
      frame 1 {
        n212 = Unbundle By Name(w336) -> ("总磷"=w335:dbl)
        n213 = global read "总磷总氮断电保存全局变量.vi" "总磷自动测试量程配置"() -> (w343:T11)
        n214 = Unbundle By Name(w341) -> ("总磷跨度值"=w340:dbl, "总磷零点标准液浓度"=w339:dbl, "总磷跨度标准液浓度"=w338:dbl, "总磷标准液标准浓度"=w337:dbl, "总磷零点标准液偏差"=w334:dbl, "总磷跨度标准液偏差"=w333:dbl, "总磷标准液标准偏差"=w332:dbl)
        n215 = global read "总磷总氮断电保存全局变量.vi" "总磷消解时长"() -> (w342:dbl)
      }
      frame 2 {
        n216 = Unbundle By Name(w348) -> ("总氮"=w347:dbl)
        n217 = global read "总磷总氮断电保存全局变量.vi" "总氮自动测试量程配置"() -> (w355:T11)
        n218 = Unbundle By Name(w353) -> ("总氮跨度值"=w352:dbl, "总氮零点标准液浓度"=w351:dbl, "总氮跨度标准液浓度"=w350:dbl, "总氮标准液标准浓度"=w349:dbl, "总氮零点标准液偏差"=w346:dbl, "总氮跨度标准液偏差"=w345:dbl, "总氮标准液标准偏差"=w344:dbl)
        n219 = global read "总磷总氮断电保存全局变量.vi" "总氮消解时长"() -> (w354:dbl)
      }
      frame 3 {
        n220 = Unbundle By Name(w360) -> ("氨氮"=w359:dbl)
        n221 = global read "总磷总氮断电保存全局变量.vi" "氨氮自动测试量程配置"() -> (w366:T11)
        n222 = Unbundle By Name(w365) -> ("氨氮跨度值"=w364:dbl, "氨氮零点标准液浓度"=w363:dbl, "氨氮跨度标准液浓度"=w362:dbl, "氨氮标准液标准浓度"=w361:dbl, "氨氮零点标准液偏差"=w358:dbl, "氨氮跨度标准液偏差"=w357:dbl, "氨氮标准液标准偏差"=w356:dbl)
      }
      frame 4 {
        n223 = Unbundle By Name(w371) -> ("磷酸盐"=w370:dbl)
        n224 = global read "总磷总氮断电保存全局变量.vi" "磷酸盐自动测试量程配置"() -> (w377:T11)
        n225 = Unbundle By Name(w376) -> ("磷酸盐跨度值"=w375:dbl, "磷酸盐零点标准液浓度"=w374:dbl, "磷酸盐跨度标准液浓度"=w373:dbl, "磷酸盐标准液标准浓度"=w372:dbl, "磷酸盐零点标准液偏差"=w369:dbl, "磷酸盐跨度标准液偏差"=w368:dbl, "磷酸盐标准液标准偏差"=w367:dbl)
      }
      frame 5 {
        n226 = Unbundle By Name(w382) -> ("硝氮"=w381:dbl)
        n227 = global read "总磷总氮断电保存全局变量.vi" "硝氮自动测试量程配置"() -> (w388:T11)
        n228 = Unbundle By Name(w387) -> ("硝氮跨度值"=w386:dbl, "硝氮零点标准液浓度"=w385:dbl, "硝氮跨度标准液浓度"=w384:dbl, "硝氮标准液标准浓度"=w383:dbl, "硝氮零点标准液偏差"=w380:dbl, "硝氮跨度标准液偏差"=w379:dbl, "硝氮标准液标准偏差"=w378:dbl)
      }
      frame 6 {
        n229 = Unbundle By Name(w393) -> ("亚硝氮"=w392:dbl)
        n230 = global read "总磷总氮断电保存全局变量.vi" "亚硝氮自动测试量程配置"() -> (w399:T11)
        n231 = Unbundle By Name(w398) -> ("亚硝氮跨度值"=w397:dbl, "亚硝氮零点标准液浓度"=w396:dbl, "亚硝氮跨度标准液浓度"=w395:dbl, "亚硝氮标准液标准浓度"=w394:dbl, "亚硝氮零点标准液偏差"=w391:dbl, "亚硝氮跨度标准液偏差"=w390:dbl, "亚硝氮标准液标准偏差"=w389:dbl)
      }
      frame 7 {
        n232 = Unbundle By Name(w404) -> ("硅酸盐"=w403:dbl)
        n233 = global read "总磷总氮断电保存全局变量.vi" "硅酸盐自动测试量程配置"() -> (w410:T11)
        n234 = Unbundle By Name(w409) -> ("硅酸盐跨度值"=w408:dbl, "硅酸盐零点标准液浓度"=w407:dbl, "硅酸盐跨度标准液浓度"=w406:dbl, "硅酸盐标准液标准浓度"=w405:dbl, "硅酸盐零点标准液偏差"=w402:dbl, "硅酸盐跨度标准液偏差"=w401:dbl, "硅酸盐标准液标准偏差"=w400:dbl)
      }
      frame 8 {
        n235 = Unbundle By Name(w415) -> ("硫化物"=w414:dbl)
        n236 = global read "总磷总氮断电保存全局变量.vi" "硫化物自动测试量程配置"() -> (w421:T11)
        n237 = Unbundle By Name(w420) -> ("硫化物跨度值"=w419:dbl, "硫化物零点标准液浓度"=w418:dbl, "硫化物跨度标准液浓度"=w417:dbl, "硫化物标准液标准浓度"=w416:dbl, "硫化物零点标准液偏差"=w413:dbl, "硫化物跨度标准液偏差"=w412:dbl, "硫化物标准液标准偏差"=w411:dbl)
      }
      frame 22 {
        n238 = Unbundle By Name(w426) -> ("COD"=w425:dbl)
        n239 = global read "总磷总氮断电保存全局变量.vi" "COD自动测试量程配置"() -> (w433:T11)
        n240 = Unbundle By Name(w431) -> ("COD跨度值"=w430:dbl, "COD零点标准液浓度"=w429:dbl, "COD跨度标准液浓度"=w428:dbl, "COD标准液标准浓度"=w427:dbl, "COD零点标准液偏差"=w424:dbl, "COD跨度标准液偏差"=w423:dbl, "COD标准液标准偏差"=w422:dbl)
        n241 = global read "总磷总氮断电保存全局变量.vi" "CODcr消解时长"() -> (w432:dbl)
      }
      frame 50 {
        n242 = Unbundle By Name(w438) -> ("氟化物"=w437:dbl)
        n243 = global read "总磷总氮断电保存全局变量.vi" "氟化物自动测试量程配置"() -> (w444:T11)
        n244 = Unbundle By Name(w443) -> ("氟化物跨度值"=w442:dbl, "氟化物零点标准液浓度"=w441:dbl, "氟化物跨度标准液浓度"=w440:dbl, "氟化物标准液标准浓度"=w439:dbl, "氟化物零点标准液偏差"=w436:dbl, "氟化物跨度标准液偏差"=w435:dbl, "氟化物标准液标准偏差"=w434:dbl)
      }
    }
    "消解时长" <- w317
    "低量程上限" <- w305
    n245 = local write "标样核查自动补测"(w300) -> ()
    n246 = local write "跨度值"(w319) -> ()
    n247 = local write "零点核查标液浓度"(w320) -> ()
    n248 = local write "跨度核查标液浓度"(w321) -> ()
    n249 = local write "标样核查标液浓度"(w322) -> ()
    n250 = local write "零点核查标液偏差"(w304) -> ()
    n251 = local write "跨度核查标液偏差"(w303) -> ()
    n252 = local write "标样核查标液偏差"(w302) -> ()
    n253 = To Unsigned Word Integer(number=w316) -> (unsigned 16bit integer=w315:T12)
    n254 = Unbundle By Name(w315) -> ("水样测试量程模式"=w314:u16, "空白核查量程模式"=w312:u16, "跨度核查量程模式"=w311:u16, "加标回收量程模式"=w310:u16, "标样核查量程模式"=w313:u16)
    n255 = local write "水样测试量程模式"(w314) -> ()
    n256 = local write "零点核查量程模式"(w312) -> ()
    n257 = local write "跨度核查量程模式"(w311) -> ()
    n258 = local write "加标回收量程模式"(w310) -> ()
    n259 = local write "标样核查量程模式"(w313) -> ()
  }
  n260 = while {
    tunnel: w2 -> [w455]
    tunnel: w3 -> [w454]
    tunnel: w4 -> [w453]
    tunnel: w1 -> [w452]
    stop <- FALSE stop-if-true
    n261 = Wait on Occurrence(2:w452) -> (0:w446:bool)  [unwired: 2 in]
    n262 = flat-sequence {
      tunnel: w455 -> [w462]
      tunnel: w454 -> [w461]
      tunnel: w453 -> [w460]
      tunnel: [w459] -> w449
      tunnel: [w458] -> w448
      tunnel: [w457] -> w447
      tunnel: w446 -> [_]
      frame #0 {
        n263 = property class="Enum (严格)"(reference=w460) -> ("Value"=w457:T1)  [unwired: 1 in, 2 out]
        n264 = property class="Enum (严格)"(reference=w461) -> ("Value"=w458:enum16{"低量程", "高量程"})  [unwired: 1 in, 2 out]
        n265 = property class="Ring (严格)"(reference=w462) -> ("Value"=w459:u16)  [unwired: 1 in, 2 out]
      }
    }
    n266 = flat-sequence {
      tunnel: [w465] -> w451
      tunnel: [w464] -> w450
      tunnel: w449 -> [w463]
      tunnel: w448 -> [w465]
      tunnel: w447 -> [w464]
      tunnel: [w463] -> w445
      tunnel: w451 -> [w484]
      tunnel: w450 -> [w485]
      tunnel: w445 -> [w483]
      frame #0 {
      }
      frame #1 {
        n267 = call "总磷总氮量程读取.vi"("测量参数"=w483) -> ("error out"=w474:errorcluster, "量程参数读取"=w482:T5)  [unwired: 9 in]
        n268 = Unbundle By Name(w482) -> ("测量精度"=→"测量精度":u16, "检出限"=→"检出限":dbl, "上限"=→"高量程上限":dbl, "下限"=→"量程下限":dbl, "阈值（低->高）"=→"阈值（低->高）":dbl, "阈值（高->低）"=→"阈值（高->低）":dbl, "稀释度"=→"稀释度":dbl)
        n269 = global read "VAR总磷总氮全局变量.vi" "MB session in"() -> (w467:refnum<class "MB_Master.lvclass">)
        n270 = call "总磷总氮公式读取.vi"("error in (no error)"=w474, "量程"=w484, "测量模式"=w485, "测量参数"=w483) -> ("error out"=w468:errorcluster, "公式"=w473:cluster{"X^2":dbl, "X":dbl, "b":dbl})  [unwired: 6 in]
        n271 = case shown="0, 默认" w483 {
          tunnel: [_ w493] -> w469
          tunnel: [w486 w489] -> _
          tunnel: w468 -> [w486 w492]
          tunnel: w467 -> [_ w491]
          tunnel: [_ w487] -> w466
          frame 0, Default {
          }
          frame 1, 2, 22 {
            n272 = call "读取外设配置.vi"("error in (no error)"=w492, "MB session in"=w491) -> ("error out"=w490:errorcluster, "外设配置"=w494:T6, "MB session out"=w488:refnum<class "MB_Master.lvclass">)  [unwired: 7 in]
            n273 = Unbundle By Name(w494) -> ("消解温度下限"=w493:sgl)
            n274 = call "盐度补偿值读取.vi"("Error in"=w490, "MB session in"=w488) -> ("error out"=w489:errorcluster, "盐度补偿值"=w487:sgl)  [unwired: 7 in, 1 out]
          }
        }
        "消解温度" <- w469
        "盐度补偿值" <- w466
        n275 = Unbundle By Name(w473) -> ("X^2"=→"二次多项式系数":dbl, "X"=→"曲线斜率":dbl, "b"=→"曲线截距":dbl)
      }
      frame #2 {
        n276 = Format Date/Time String() -> (date/time string=→"数据刷新时间":string)  [unwired: 3 in]
      }
    }
  }
